vi "genRVCtrajTL.vi"() -> ()   [LabVIEW 2016]
uses:
  <vilib>/Math Plots/3D Math Plots/3D Scatter/3D Scatter XCtrl/3D Scatter.xctl
  <vilib>/Analysis/1siggen.llb/Ramp Pattern by Samples.vi
  Subsystems/Global Variables.vi
  <vilib>/Math Plots/3D Math Plots/3D Scatter/3D Scatter Datatype/Public/Plot Helper (Vector).vi
  <vilib>/Math Plots/3D Math Plots/3D Scatter/3D Scatter Datatype/3D Scatter Datatype.lvclass
  <vilib>/gmath/NI_Gmath.lvlib
  <vilib>/Analysis/NI_AALBase.lvlib
  <vilib>/Utility/file.llb/Read Delimited Spreadsheet (DBL).vi
panel:
  out "DH Params":cluster{"d_DH":dbl[][], "ty":dbl[][]}
  out "J3 Array":dbl[](array[numeric])
  out "J2 Array":dbl[](array[numeric])
  out "J1 Array":dbl[](array[numeric])
  in  "offsetZ":dbl
  in  "offsetX":dbl
  in  "offsetY":dbl
  out "size(s)":i32
  out "zVisTraj":dbl[](array[numeric]) format="%_6g"
  out "yVisTraj":dbl[](array[numeric]) format="%_6g"
  out "xVisTraj":dbl[](array[numeric]) format="%_6g"
  out "Traj Plot":refnum<class "3D Plot Datatype.lvclass">[](xcontrol)
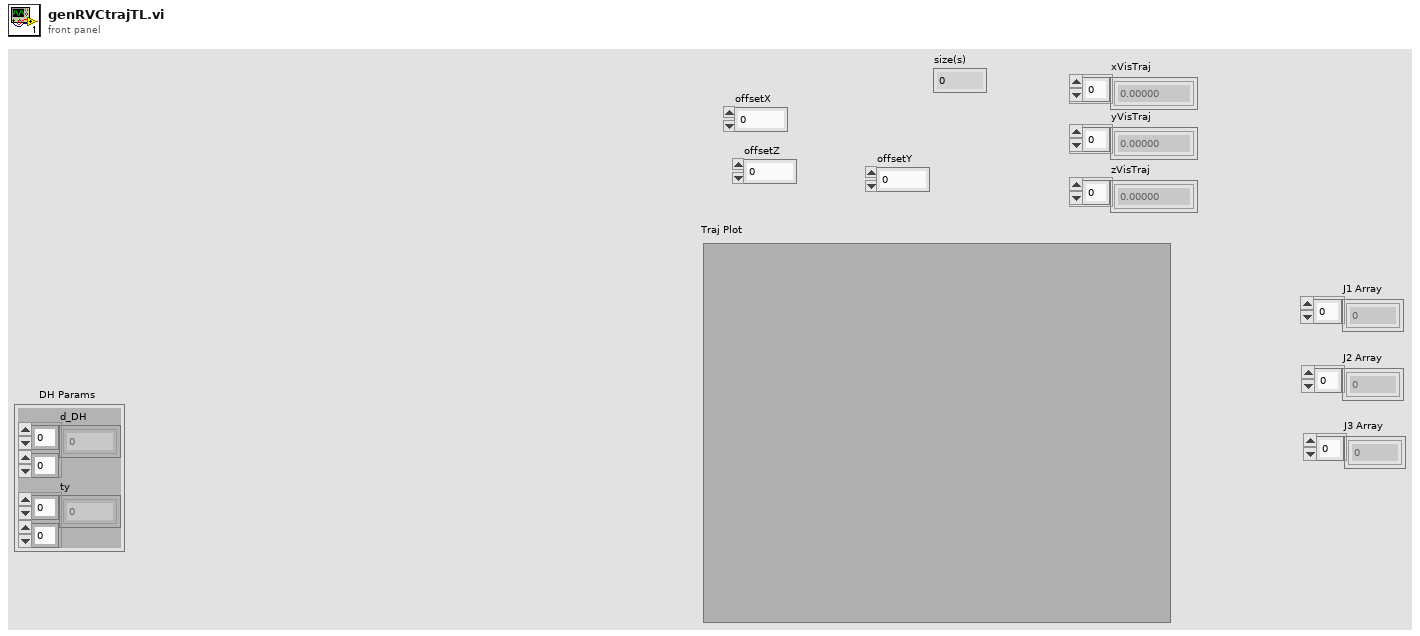
[diagram p1: front panel]
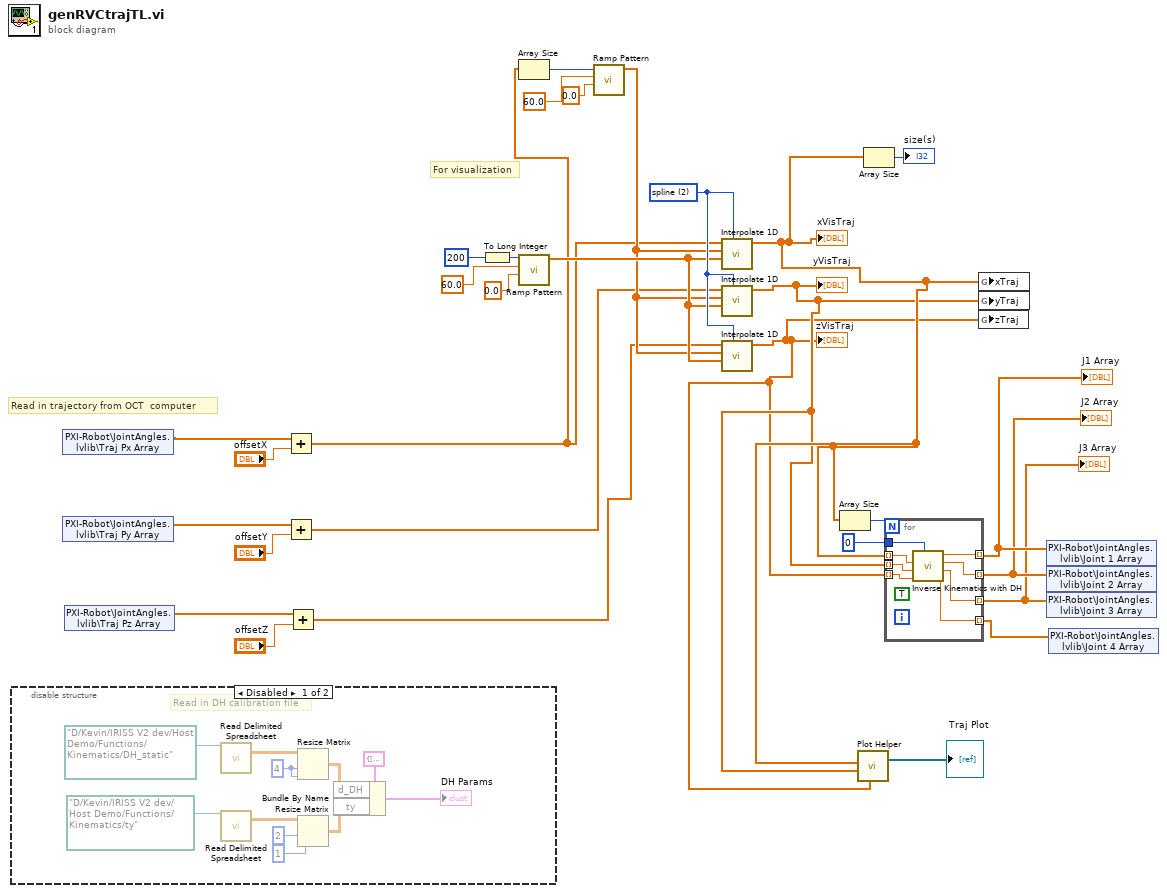
[diagram p0: block diagram]
diagram:
  w30 = 2 items=["nearest", "linear", "spline", "cubic Hermite", "Lagrange"] ("method")
  # "Read in trajectory from OCT  computer"
  # "For visualization"
  n1 = disable-structure shown="Disabled" {
    frame Disabled {
      w39 = 4 ("number of rows")
      # "Read in DH calibration file"
      n2 = call-poly <vilib>:"Read Delimited Spreadsheet.vi"("file path (dialog if empty)"=path "D:/Kevin/IRISS V2 dev/Host Demo/Functions/Kinematics/DH_static" ("file path (use dialog)")) -> ("all rows"=w40:dbl[][])  [unwired: 9 in, 5 out]
      n3 = call-poly <vilib>:"Read Delimited Spreadsheet.vi"("file path (dialog if empty)"=path "D:/Kevin/IRISS V2 dev/Host Demo/Functions/Kinematics/ty" ("file path (use dialog)")) -> ("all rows"=w38:dbl[][])  [unwired: 9 in, 5 out]
      n4 = Resize Matrix(1:w39, 2:w39, 4:w40) -> (0:w34:dbl[][])
      n5 = Resize Matrix(1:1 ("number of columns"), 2:2 ("number of rows"), 4:w38) -> (0:w33:dbl[][])
      n6 = Bundle By Name(cluster=cluster{"d_DH":dbl[][], "ty":dbl[][]} {"d_DH"=[[0.0, -0.04858099004841317, 1.1971672750675049, 0.0], [0.0, -1.576475511297109, 0.0, 0.0], [-0.3552491783526254, 0.0, -1.1064589410656984, 0.2058446720735121], [-1.0573457532495087, 1.0278049025155533, 0.011917110633363169, -0.004023577880993236]], "ty"=[[0.04320445582455471], [0.011728642746432275]]} ("input cluster"), "d_DH"=w34, "ty"=w33) -> (→"DH Params":cluster{"d_DH":dbl[][], "ty":dbl[][]})
    }
    frame Enabled {
    }
  }
  n7 = shared-variable "PXI-Robot\\JointAngles.lvlib\\Traj Px Array"() -> (w7:dbl[])  [unwired: 1 in, 1 out]
  n8 = shared-variable "PXI-Robot\\JointAngles.lvlib\\Traj Py Array"() -> (w6:dbl[])  [unwired: 1 in, 1 out]
  n9 = shared-variable "PXI-Robot\\JointAngles.lvlib\\Traj Pz Array"() -> (w5:dbl[])  [unwired: 1 in, 1 out]
  n10 = Add(x=w7, y="offsetX") -> (x+y=w13:dbl[])
  n11 = Add(x=w6, y="offsetY") -> (x+y=w8:dbl[])
  n12 = Add(x=w5, y="offsetZ") -> (x+y=w12:dbl[])
  n13 = To Long Integer(number=200) -> (32bit integer=w29:i32)
  n14 = Array Size(array=w13) -> (size(s)=w23:i32)
  n15 = call-poly <vilib>:"Ramp Pattern.vi"("start"=0.0, "end"=60.0, "samples"=w29) -> ("Ramp Pattern"=w27:dbl[])  [unwired: 7 in, 1 out]
  n16 = call-poly <vilib>:"Ramp Pattern.vi"("start"=0.0, "end"=60.0, "samples"=w23) -> ("Ramp Pattern"=w22:dbl[])  [unwired: 7 in, 1 out]
  n17 = call <vilib>:"Interpolate 1D.vi"("method"=w30, "xi"=w27, "X"=w22, "Y"=w13) -> ("yi"=w3:dbl[])  [unwired: 5 in, 2 out]
  "xVisTraj" <- w3
  n18 = call <vilib>:"Interpolate 1D.vi"("method"=w30, "xi"=w27, "X"=w22, "Y"=w8) -> ("yi"=w2:dbl[])  [unwired: 5 in, 2 out]
  "yVisTraj" <- w2
  n19 = call <vilib>:"Interpolate 1D.vi"("method"=w30, "xi"=w27, "X"=w22, "Y"=w12) -> ("yi"=w1:dbl[])  [unwired: 5 in, 2 out]
  "zVisTraj" <- w1
  n20 = Array Size(array=w3) -> (size(s)=w19:i32)
  n21 = call-poly <vilib>:"Plot Helper.vi"("z vector"=w1, "y vector"=w2, "x vector"=w3) -> ("3D Plot lvclass Array out"=→"Traj Plot":refnum<class "3D Plot Datatype.lvclass">[])  [unwired: 3 in, 5 out]
  n22 = Array Size(array=w3) -> (size(s)=→"size(s)":i32)
  n23 = for {
    N: w19 -> [_]
    tunnel: 0 ("Arm ID Ind") -> [w49]
    tunnel: w3 -> [w48] mode=indexing
    tunnel: w2 -> [w47] mode=indexing
    tunnel: w1 -> [w46] mode=indexing
    tunnel: [w43] -> w11 mode=indexing
    tunnel: [w44] -> w10 mode=indexing
    tunnel: [w45] -> w9 mode=indexing
    tunnel: [w42] -> w4 mode=indexing
    (unwired) TRUE ("isToolTipInsideEye")
    n24 = call "Inverse Kinematics with DH.vi"("armID"=w49, "z"=w46, "y"=w47, "x"=w48) -> ("j4"=w42:dbl, "j3"=w45:dbl, "j2"=w44:dbl, "j1"=w43:dbl)  [unwired: 4 in]
  }
  "J1 Array" <- w11
  "J2 Array" <- w10
  "J3 Array" <- w9
  n25 = global write "Global Variables.vi" "xTraj"(w3) -> ()
  n26 = global write "Global Variables.vi" "yTraj"(w2) -> ()
  n27 = global write "Global Variables.vi" "zTraj"(w1) -> ()
  n28 = shared-variable "PXI-Robot\\JointAngles.lvlib\\Joint 1 Array"(w11) -> ()  [unwired: 1 in, 1 out]
  n29 = shared-variable "PXI-Robot\\JointAngles.lvlib\\Joint 2 Array"(w10) -> ()  [unwired: 1 in, 1 out]
  n30 = shared-variable "PXI-Robot\\JointAngles.lvlib\\Joint 3 Array"(w9) -> ()  [unwired: 1 in, 1 out]
  n31 = shared-variable "PXI-Robot\\JointAngles.lvlib\\Joint 4 Array"(w4) -> ()  [unwired: 1 in, 1 out]
